vi "pmu_Read Performance Class.vi"(8 "error in (no error)":errorcluster, 11 "system info in":refnum<class "PMU System Info.lvclass">) -> (0 "error out":errorcluster, 2 "performance class":enum8{"M Class", "P Class"}(ring), 3 "system info out":refnum<class "PMU System Info.lvclass">)   [LabVIEW 2013, in "NI_EP_PMU.lvlib" / "PMU System Info.lvclass"]
uses:
  <vilib>/addons/Electrical Power/PMU/Common/Classes/PMU System Info/PMU System Info.lvclass
  <vilib>/addons/Electrical Power/PMU/Common/Classes/PMU System Info/PMU System Info.lvclass/PMU System Info.ctl
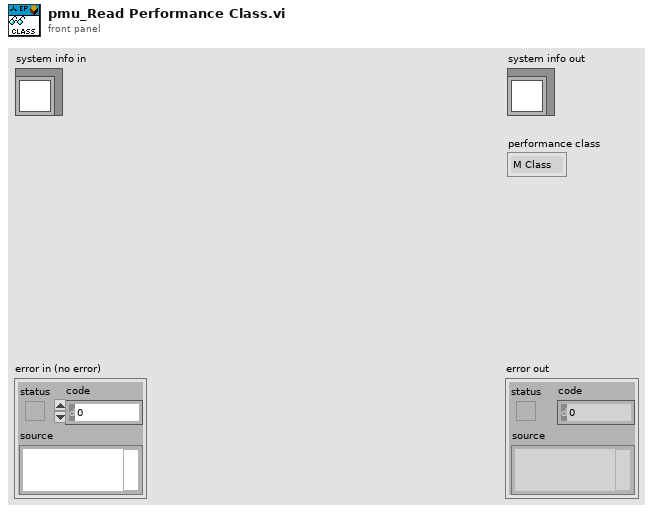
[diagram p1: front panel]
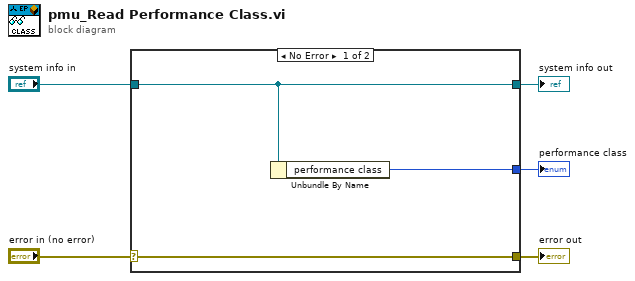
[diagram p0: block diagram]
diagram:
  n1 = case shown="No Error" "error in (no error)" {
    selector: "error in (no error)" -> [w8 w9]
    tunnel: [w8 w9] -> w4
    tunnel: [w7 w10] -> w2
    tunnel: "system info in" -> [w7 w10]
    tunnel: [w6 _] -> w1
    frame No Error {
      n2 = Unbundle By Name(w7) -> ("performance class"=w6:enum8{"M Class", "P Class"})
    }
    frame Error {
    }
  }
  "error out" <- w4
  "system info out" <- w2
  "performance class" <- w1
